vi "sendSignal.vi"(8 "error in (no error)":errorcluster, 10 "Throttle [%]":dbl, 11 "Exceed RC Volcano Series in":refnum<class "Exceed RC Volcano Series.lvclass">) -> (0 "error out":errorcluster, 3 "Exceed RC Volcano Series out":refnum<class "Exceed RC Volcano Series.lvclass">)   [LabVIEW 2015, in "Exceed RC Volcano Series.lvclass"]
uses:
  Exceed RC Volcano Series.lvclass
  Exceed RC Volcano Series.lvclass/Exceed RC Volcano Series.ctl
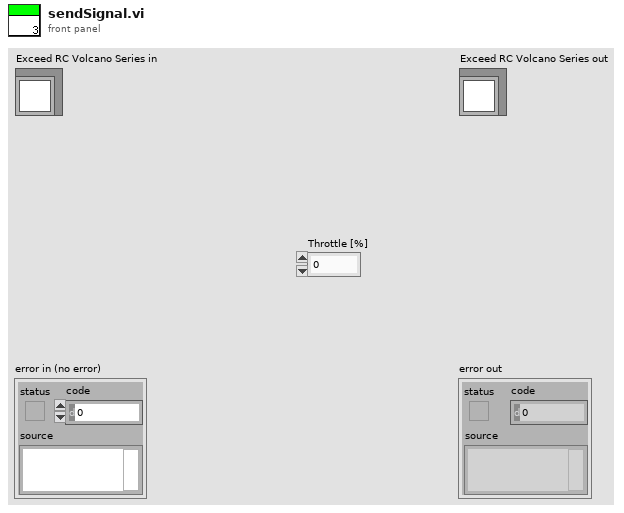
[diagram p1: front panel]
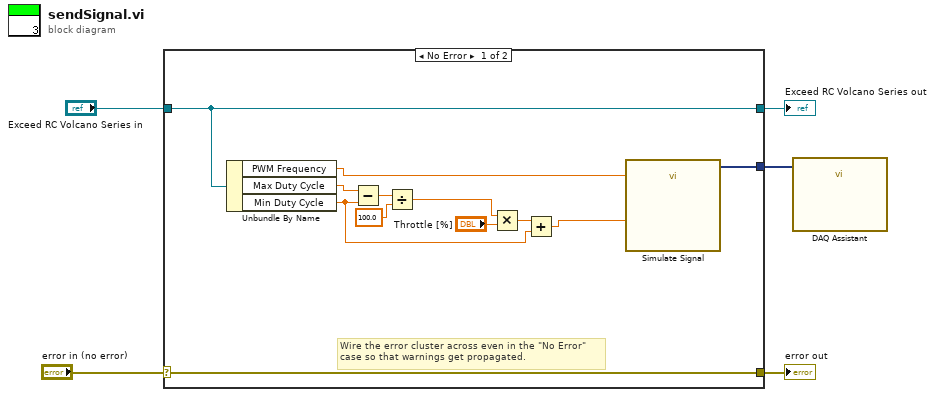
[diagram p0: block diagram]
diagram:
  n1 = case shown="No Error" "error in (no error)" {
    selector: "error in (no error)" -> [w17 w19]
    tunnel: [w17 w19] -> w4
    tunnel: [w7 w18] -> w2
    tunnel: "Exceed RC Volcano Series in" -> [w7 w18]
    tunnel: [w6 _] -> w1
    frame No Error {
      # "Wire the error cluster across even in the \"No Error\"\ncase so that warnings get propagated."
      n2 = Unbundle By Name(w7) -> ("PWM Frequency"=w13:dbl, "Max Duty Cycle"=w12:dbl, "Min Duty Cycle"=w15:dbl)
      n3 = Subtract(x=w12, y=w15) -> (x-y=w8:dbl)
      n4 = Divide(x=w8, y=100.0) -> (x/y=w11:dbl)
      n5 = Multiply(x=w11, y="Throttle [%]") -> (x*y=w14:dbl)
      n6 = Add(x=w14, y=w15) -> (x+y=w16:dbl)
      n7 = call "Simulate Signal"("Duty Cycle (%)"=w16, "Frequency"=w13) -> ("Square"=w6:dynamicdata)  [unwired: 12 in, 1 out]
    }
    frame Error {
    }
  }
  "error out" <- w4
  "Exceed RC Volcano Series out" <- w2
  n8 = call "DAQ Assistant"("data"=w1) -> ()  [unwired: 16 in, 3 out]
